vi "Read Paired Tunnels of Case Structure.vi"(8 "error in (no error)":errorcluster, 11 "CSM-Helper in":refnum<class "CSM-Helper.lvclass">) -> (0 "error out":errorcluster, 1 "Paired Tunnels":cluster{refnum<vi>, refnum<vi>}[](array[cluster]), 3 "CSM-Helper out":refnum<class "CSM-Helper.lvclass">)   [LabVIEW 2017, in "CSM-Helper.lvclass"]
doc: "### Read Paired Tunnels of Case Structure.vi\n\n-- <b>Controls</b> --\n- <b>CSM-Helper in</b>: CSMHelper input\n\n-- <b>Indicators</b> --\n- <b>Paired Tunnels</b>:\n- <b>CSM-Helper out</b>: CSMHelper output"
uses:
  CSM-Helper.lvclass
  CSM-Helper.lvclass/CSM-Helper.ctl
  Read Case Structure Ref.vi
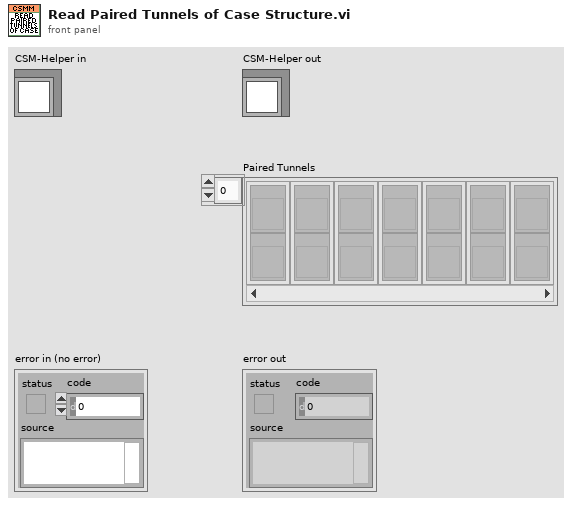
[diagram p1: front panel]
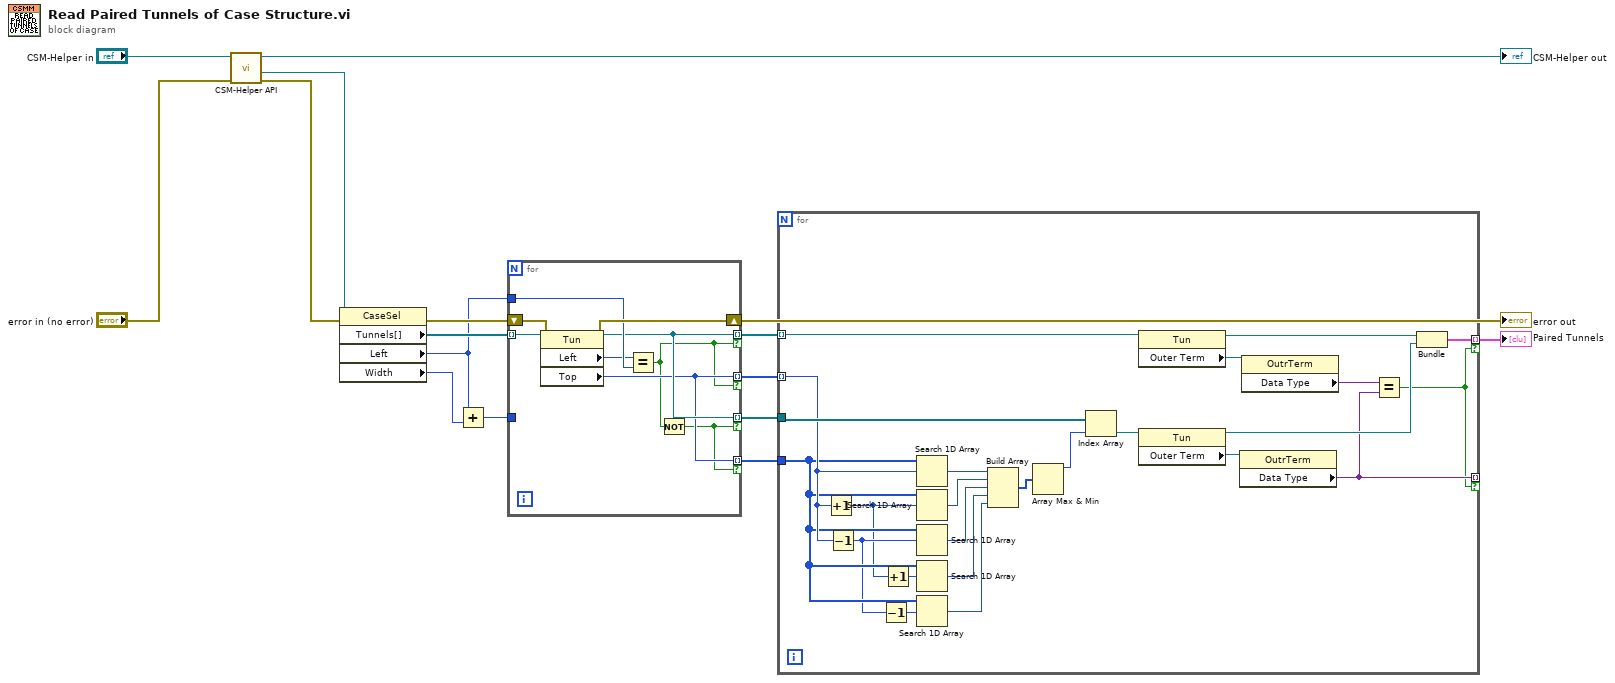
[diagram p0: block diagram]
diagram:
  n1 = call-poly "CSM-Helper API.vi"("error in (no error)"="error in (no error)", "CSM-Helper in"="CSM-Helper in") -> ("error out"=w11:errorcluster, "Case Structure"=w14:refnum<vi>, "CSM-Helper out"=→"CSM-Helper out":refnum<class "CSM-Helper.lvclass">)  [unwired: 7 in]
  n2 = property on="Property Node" class="CaseSel"(reference=w14, error in=w11) -> (error out=w10:errorcluster, "Tunnels[]"=w13:refnum<vi>[], "Left"=w7:i32, "Width"=w9:u32)  [unwired: 1 out]
  n3 = Add(x=w7, y=w9) -> (x+y=w8:u32)
  n4 = for {
    tunnel: w13 -> [w25] mode=indexing
    shift-right: [w23] -> w6
    shift-left: w10 -> [w24]
    tunnel: w8 -> [_]
    tunnel: w7 -> [w22]
    tunnel: [w21] -> w4 mode=indexing if=w17
    tunnel: [w21] -> w3 mode=indexing if=w18
    tunnel: [w19] -> w5 mode=indexing if=w17
    tunnel: [w19] -> w2 mode=indexing if=w18
    n5 = property class="Tun"(reference=w25, error in=w24) -> (reference out=w21:refnum<vi>, error out=w23:errorcluster, "Left"=w20:i32, "Top"=w19:i32)
    n6 = Equal?(x=w20, y=w22) -> (x = y?=w17:bool)
    n7 = Not(x=w17) -> (.not. x?=w18:bool)
  }
  "error out" <- w6
  n8 = for {
    tunnel: w5 -> [w38] mode=indexing
    tunnel: w4 -> [w48] mode=indexing
    tunnel: w3 -> [w49]
    tunnel: w2 -> [w30]
    tunnel: [w41] -> w1 mode=indexing if=w39
    tunnel: [w40] -> _ mode=indexing if=w39
    n9 = Increment(x=w38) -> (x+1=w28:i32)
    n10 = Decrement(x=w38) -> (x-1=w29:i32)
    n11 = Decrement(x=w29) -> (x-1=w26:i32)
    n12 = Increment(x=w28) -> (x+1=w27:i32)
    n13 = Search 1D Array(1D array=w30, element=w38) -> (index of element=w37:i32)  [unwired: 1 in]
    n14 = Search 1D Array(1D array=w30, element=w28) -> (index of element=w36:i32)  [unwired: 1 in]
    n15 = Search 1D Array(1D array=w30, element=w29) -> (index of element=w35:i32)  [unwired: 1 in]
    n16 = Search 1D Array(1D array=w30, element=w27) -> (index of element=w32:i32)  [unwired: 1 in]
    n17 = Search 1D Array(1D array=w30, element=w26) -> (index of element=w31:i32)  [unwired: 1 in]
    n18 = Build Array(w37, w36, w35, w32, w31) -> (w34:i32[])
    n19 = Array Max & Min(array=w34) -> (max value=w33:i32)  [unwired: 3 out]
    n20 = Index Array(array=w49, index=w33) -> (element=w47:refnum<vi>)
    n21 = property class="Tun"(reference=w48) -> (reference out=w43:refnum<vi>, "Outer Term"=w46:refnum<vi>)  [unwired: 1 in, 1 out]
    n22 = property class="Tun"(reference=w47) -> (reference out=w42:refnum<vi>, "Outer Term"=w45:refnum<vi>)  [unwired: 1 in, 1 out]
    n23 = property class="OutrTerm"(reference=w45) -> ("Data Type"=w40:variant)  [unwired: 1 in, 2 out]
    n24 = property class="OutrTerm"(reference=w46) -> ("Data Type"=w44:variant)  [unwired: 1 in, 2 out]
    n25 = Equal?(x=w44, y=w40) -> (x = y?=w39:bool)
    n26 = Bundle(w43, w42) -> (w41:cluster{refnum<vi>, refnum<vi>})  [unwired: 1 in]
  }
  "Paired Tunnels" <- w1
